vi "Read Device Type.vi"(8 "error in (no error)":errorcluster, 11 "Generic Device in":refnum<class "Generic Device.lvclass">) -> (0 "error out":errorcluster, 2 "Device Type":T1, 3 "Generic Device out":refnum<class "Generic Device.lvclass">)   [LabVIEW 2016, in "Generic Device.lvlib" / "Generic Device.lvclass"]
uses:
  Generic Device.lvclass
  Controls/Generic Device Type.ctl
  Generic Device.lvclass/Generic Device.ctl
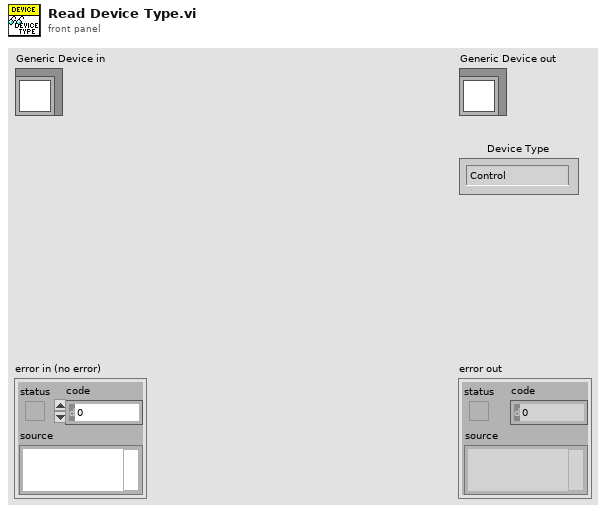
[diagram p1: front panel]
types:
  T1 = typedef "Generic Device Type.ctl" = enum16{"Control", "Instrument"}
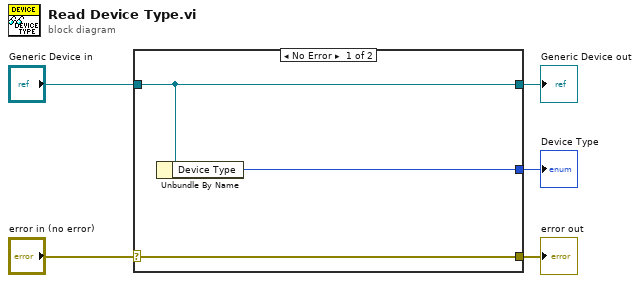
[diagram p0: block diagram]
diagram:
  n1 = case shown="No Error" "error in (no error)" {
    selector: "error in (no error)" -> [w8 w9]
    tunnel: [w8 w9] -> w4
    tunnel: [w7 w10] -> w2
    tunnel: "Generic Device in" -> [w7 w10]
    tunnel: [w6 _] -> w1
    frame No Error {
      n2 = Unbundle By Name(w7) -> ("Device Type"=w6:T1)
    }
    frame Error {
    }
  }
  "error out" <- w4
  "Generic Device out" <- w2
  "Device Type" <- w1
